vi "CheckForError.vi"(0 "Main Path":path) -> (1 "Array of Folders":path[](array[path]), 2 "PRAMMS VRN":refnum<visa-resource-name>, 3 "Array of Files":path[](array[path]), 4 "SkipInstr":bool, 6 "Bundle-Meteo":T1={"cRIO address"="0.0.0.0", "Port Number"=0, "cRIO_commID"=refnum, "Cx"=FALSE}, 8 "This VI's Path":path, 10 "term":string, 11 "Go on ?":bool, 12 "Array of Baud Rates":u32[](array[numeric]), 13 "TCS-CommVRN":refnum<visa-resource-name>, 14 "Array of VISA refnum":refnum<visa-resource-name>[](array[refnum]), 15 "Serial":bool[](array[boolean]))   [LabVIEW 2019]
uses:
  Globals.vi
  <vilib>/Utility/config.llb/Read Key (U32).vi
  <vilib>/Utility/config.llb/Read Key (String).vi
  <vilib>/Instr/_visa.llb/VISA Configure Serial Port (Instr).vi
  Comm/SerialCommError.vi
  <vilib>/Utility/config.llb/Read Key (Path).vi
  <vilib>/Utility/config.llb/NI_LVConfig.lvlib
panel:
  in  "SkipInstr":bool
  out "Hexapode":bool
  out "Hexapod VRN":refnum<visa-resource-name>
  out "PRAMMS":bool
  out "ActiveDummy":bool
  out "TCS":bool
  out "TCP Error":errorcluster
  out "standard output":string
  out "standard error":string
  out "concatenated string":string
  out "Nettoyage":bool
  in  "restart":bool
  out "error out":errorcluster
  in  "cancel":bool
  in  "ignore":bool
  out "Master Dir":path
  out "IDL":bool
  out "wget":bool
  out "Ports Series":bool
  out "SubVIs":bool
  out "config error out":errorcluster
  out "Camera":bool
  out "Starry Night":bool
  out "Configuration":bool
  out "Arborescence":bool
  # "Version sans GUI de ErrorCheck.vi  Vérifie :\n    - Existence des chemins/fichiers nécessaire\n    - Communication avec les différents périphériques\n    - Lien ActiveX avec Starry Night\n    - Vérifie la communication avec la station météo\n    - Vérifie l'état de la face avant des VIs utilisés\n    - Compatibilité des versions installées\n    - Vérifie la disponibilité des applications (wget, IDL)"
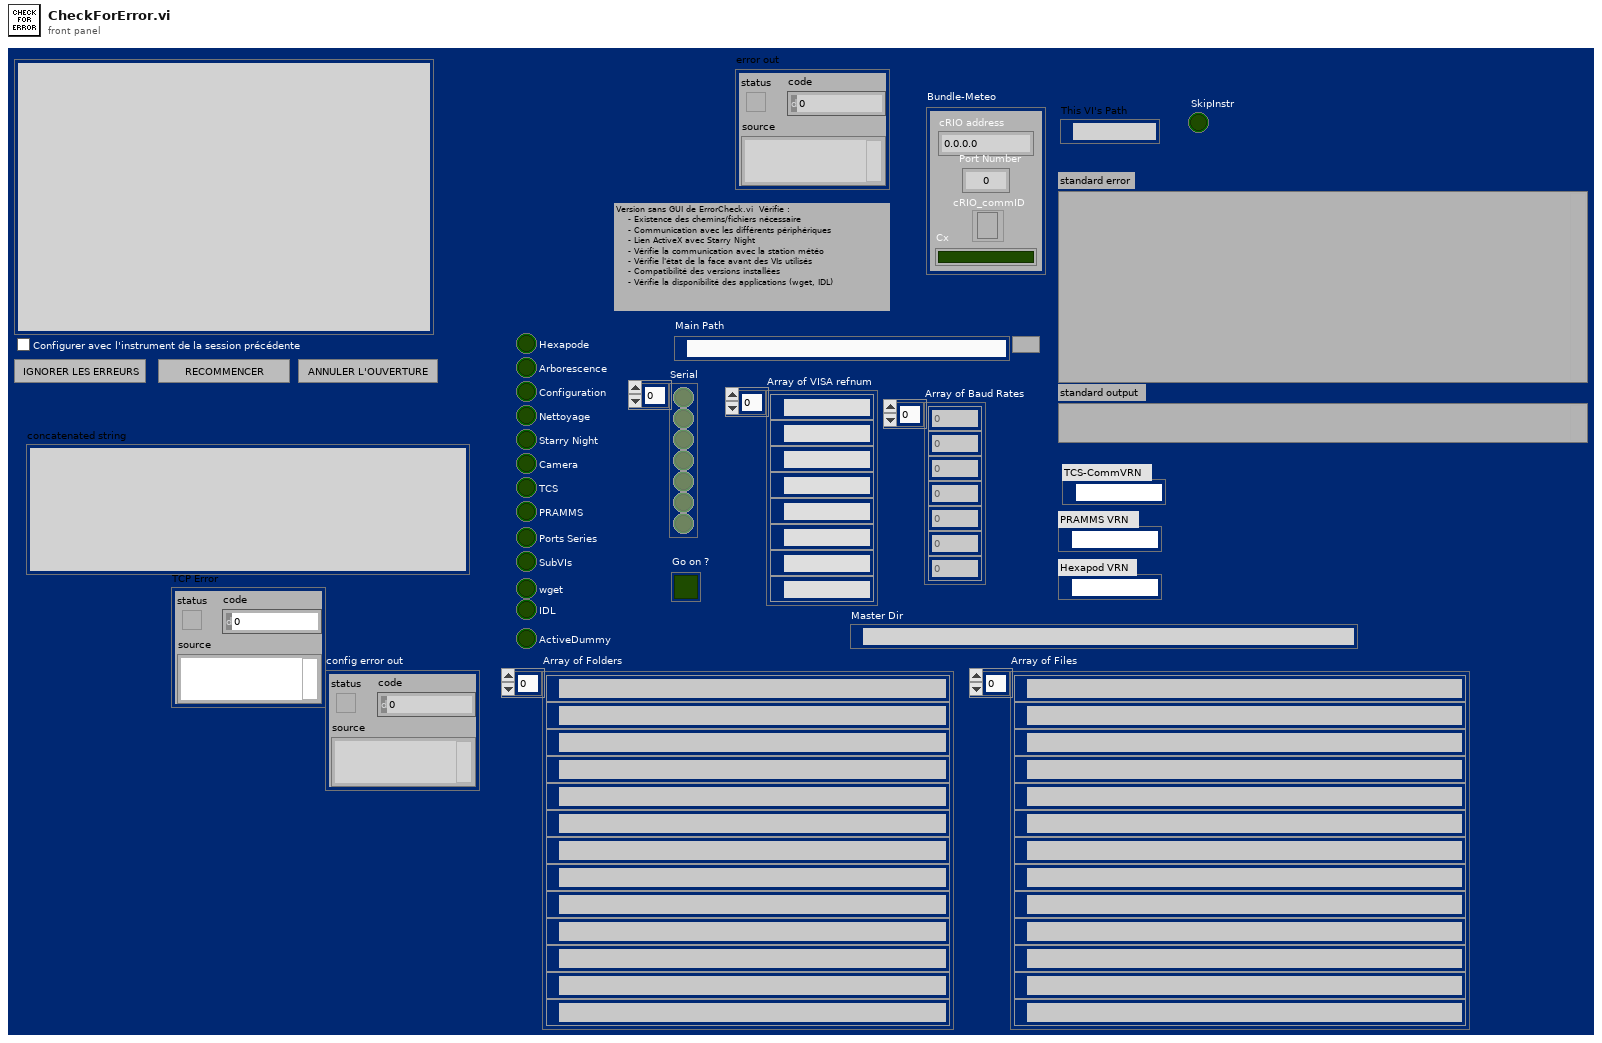
[diagram p1: front panel]
types:
  T1 = cluster{"cRIO address":string, "Port Number":u16, "cRIO_commID":refnum<k5>, "Cx":bool}
  T2 = enum8{"Enabled", "Disabled", "Disabled and Grayed Out"}
  T3 = typedef "NI_LVConfig.lvlib/Config Data RefNum.ctl" = refnum<k1>
  T4 = cluster{"value":string, u16, "connection ID":refnum<k5>, bool}
  T5 = enum16{"Left Button", "Center Button", "Right Button", "Window Close"}
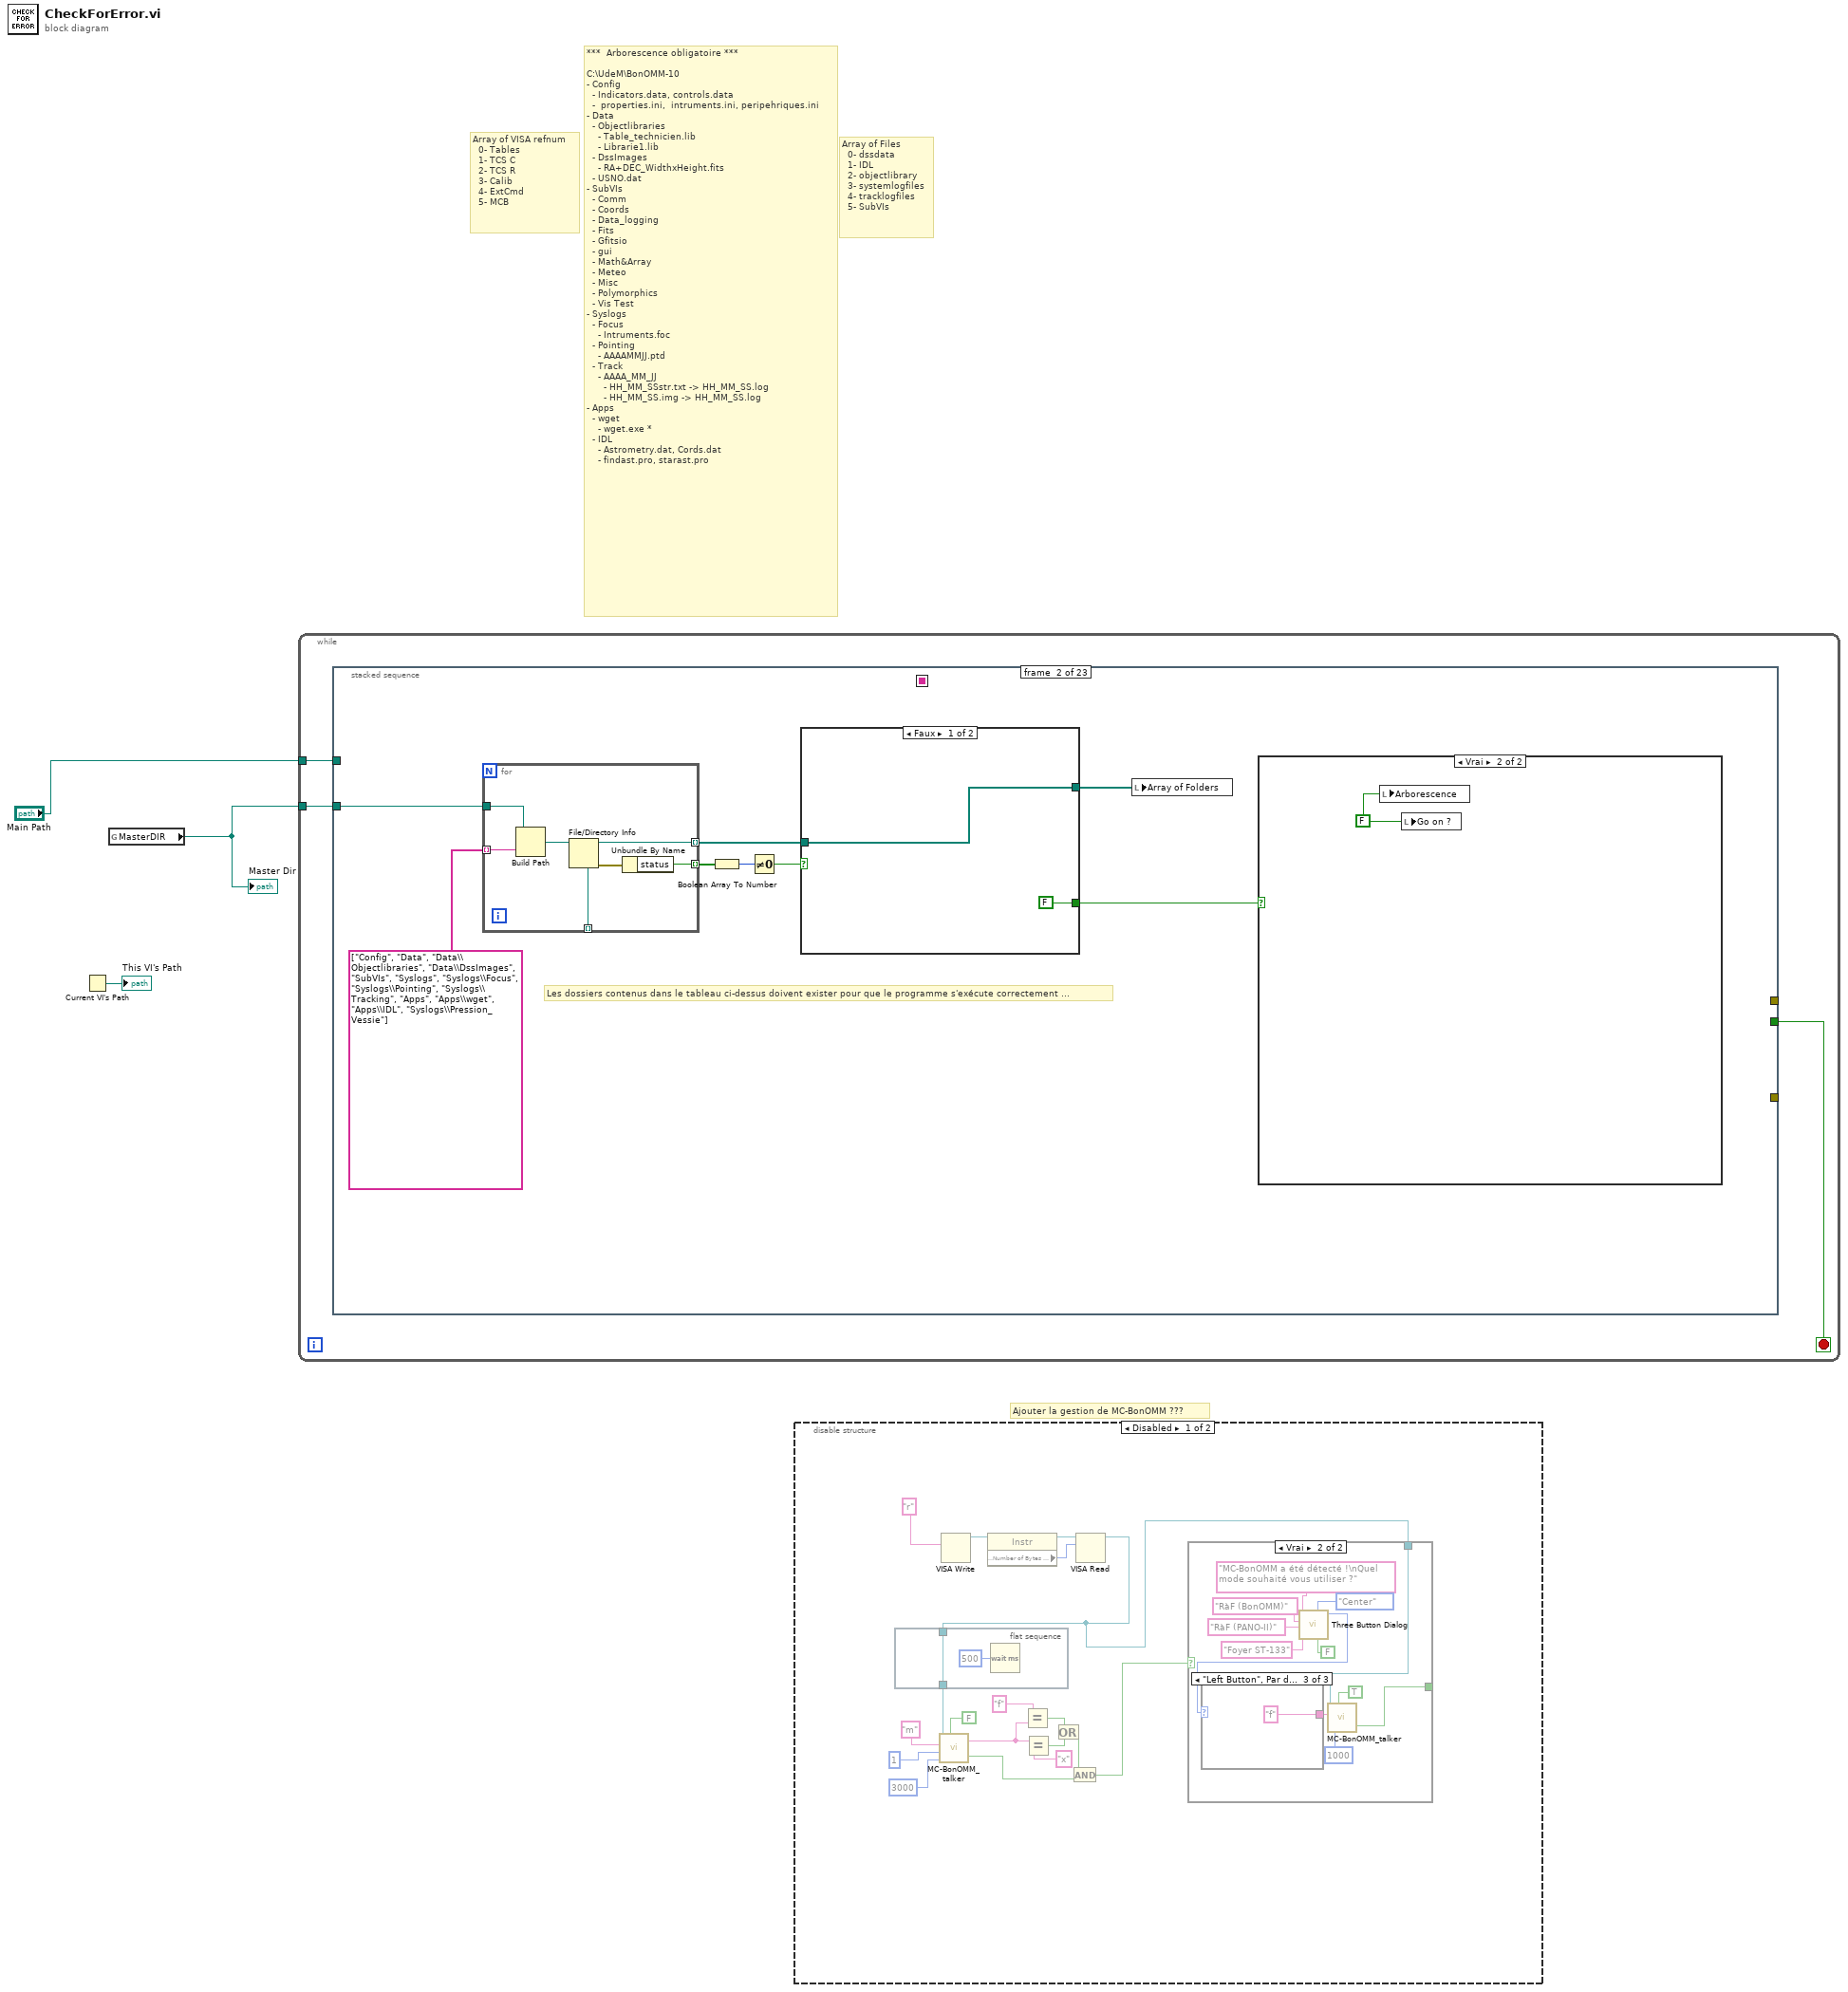
[diagram p0: block diagram]
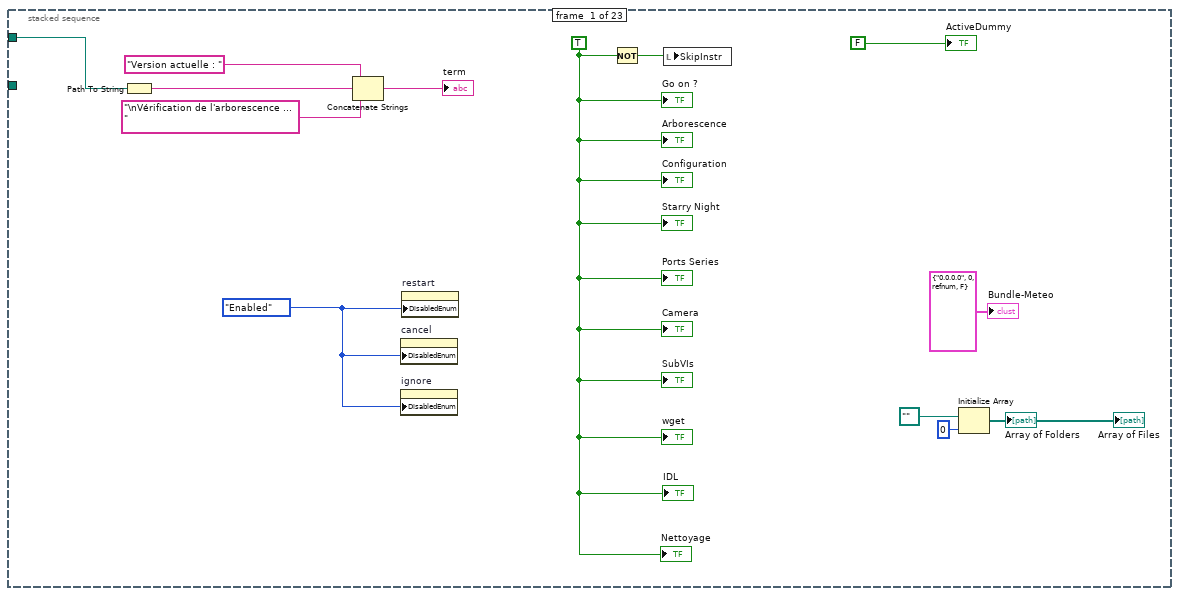
[diagram p2: hidden frame]
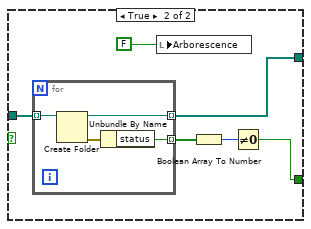
[diagram p4: hidden frame]
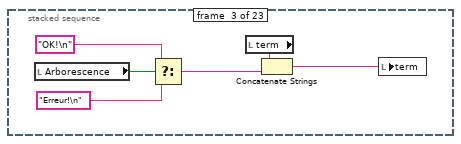
[diagram p5: hidden frame]
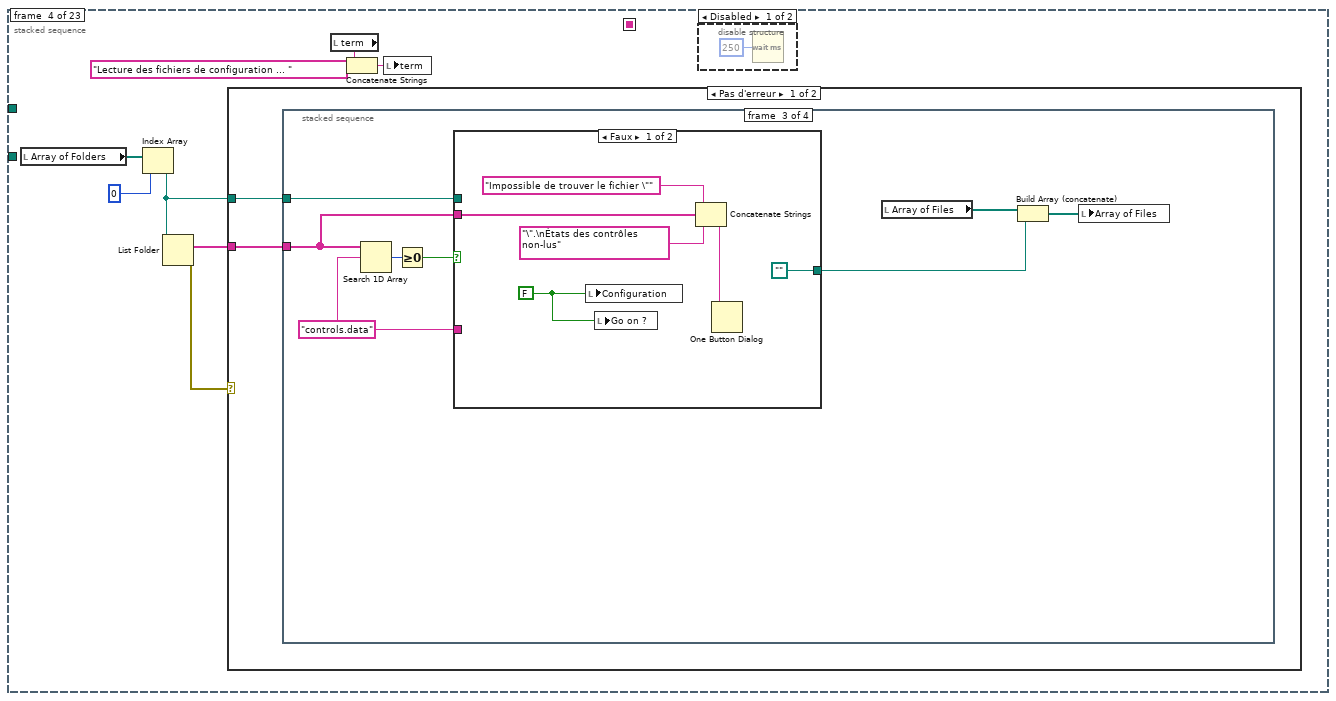
[diagram p6: hidden frame]
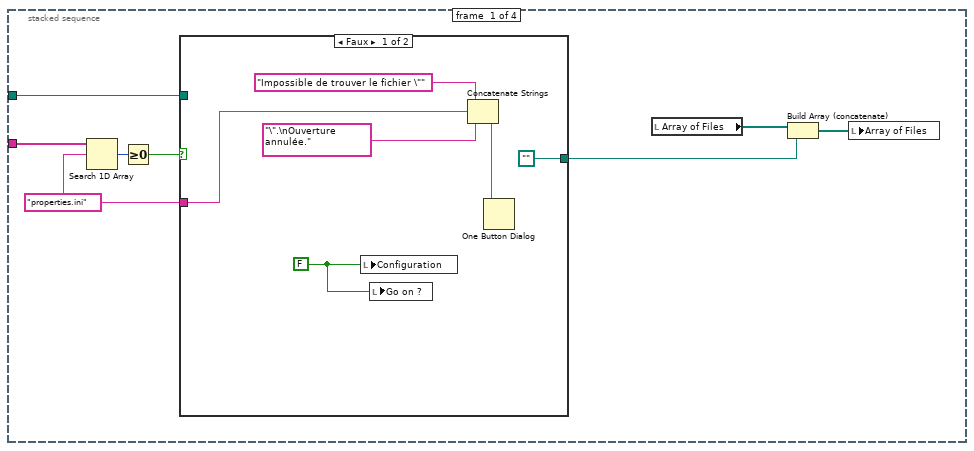
[diagram p8: hidden frame]
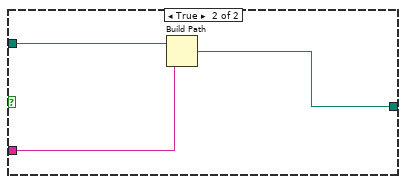
[diagram p9: hidden frame]
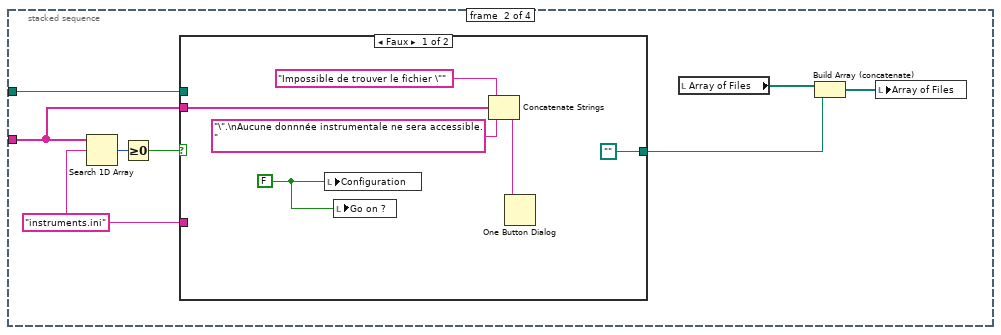
[diagram p10: hidden frame]
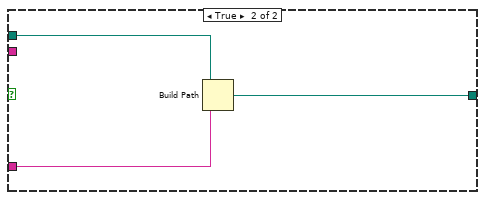
[diagram p11: hidden frame]
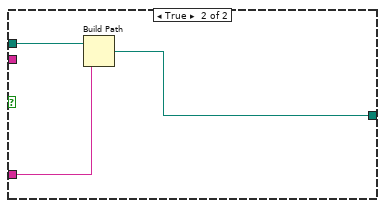
[diagram p12: hidden frame]
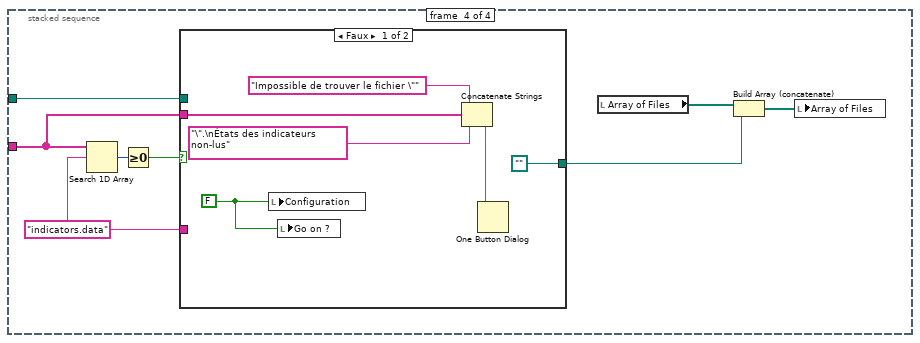
[diagram p13: hidden frame]
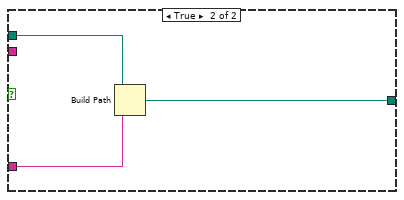
[diagram p14: hidden frame]
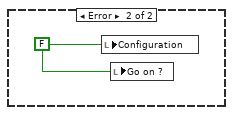
[diagram p15: hidden frame]
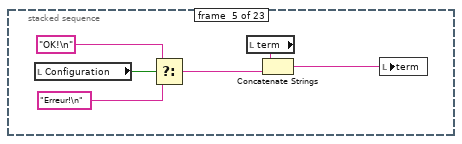
[diagram p16: hidden frame]
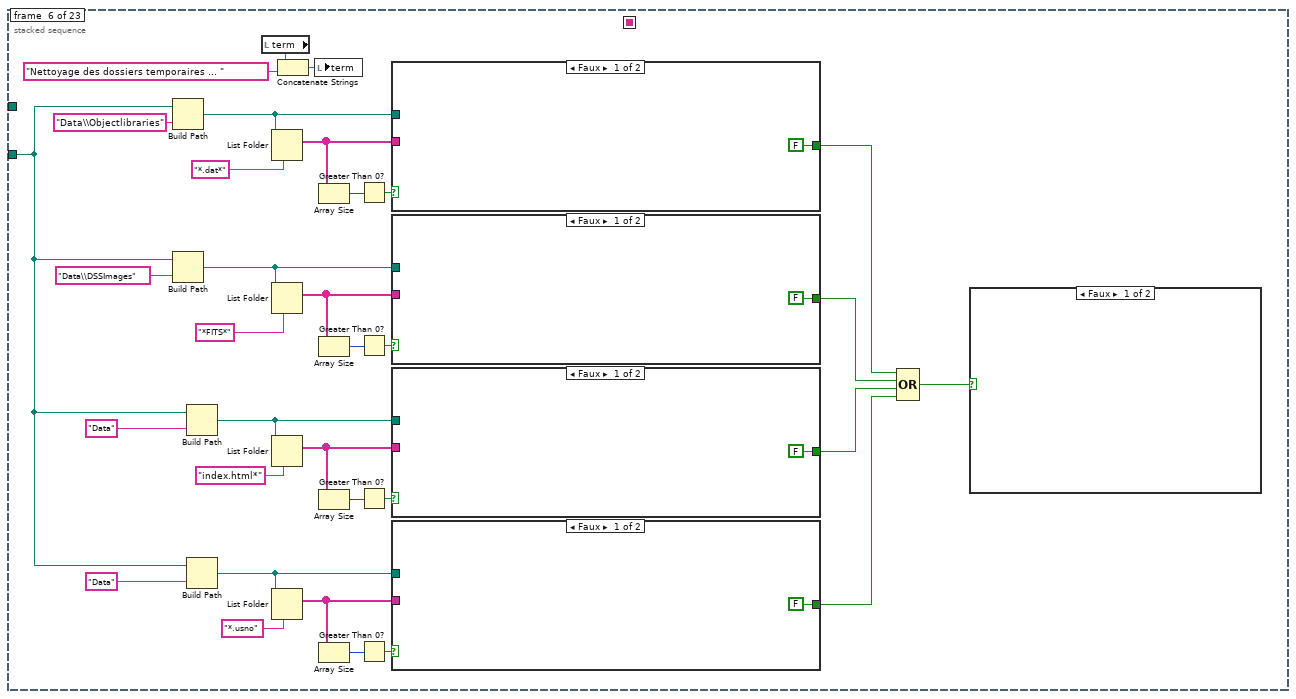
[diagram p17: hidden frame]
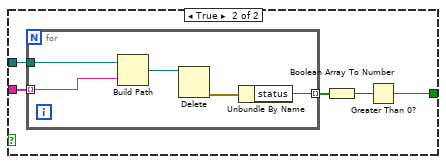
[diagram p18: hidden frame]
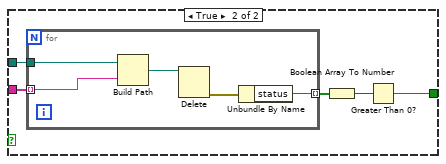
[diagram p19: hidden frame]
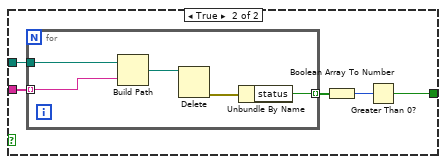
[diagram p20: hidden frame]
diagram:
  # "Array of Files\n  0- dssdata\n  1- IDL\n  2- objectlibrary\n  3- systemlogfiles\n  4- tracklogfiles\n  5- SubVIs"
  # "***  Arborescence obligatoire ***\n\nC:\\UdeM\\BonOMM-10\n-\tConfig\n  -\tIndicators.data, controls.data\n  -\t properties.ini,  intruments.ini, peripehriques.ini\n-\tData\n  -\tObjectlibraries\n    -\tTable_technicien.lib\n    -\tLibrarie1.lib\n  -\tDssImages\n    -\tRA+DEC_WidthxHeight.fits\n  -\tUSNO.dat\n-\tSubVIs\n  -\tComm\n  -\tCoords\n  -\tData_logging\n  -\tFits\n  -\tGfitsio\n  -\tgui\n  -\tMath&Array\n  -\tMeteo\n  -\tMisc\n  -\tPolymorphics\n  -\tVis Test\n-\tSyslogs\n  -\tFocus\n    -\tIntruments.foc\n  -\tPointing\n    -\tAAAAMMJJ.ptd\n  -\tTrack\n    -\tAAAA_MM_JJ\n      -\tHH_MM_SSstr.txt -> HH_MM_SS.log\n      -\tHH_MM_SS.img -> HH_MM_SS.log\n-\tApps\n  -\twget\n    -\twget.exe *\n  -\tIDL\n    -\tAstrometry.dat, Cords.dat\n    -\tfindast.pro, starast.pro"
  # "Array of VISA refnum\n  0- Tables\n  1- TCS C\n  2- TCS R\n  3- Calib\n  4- ExtCmd\n  5- MCB"
  # "Ajouter la gestion de MC-BonOMM ???"
  n1 = Current VI's Path() -> (path=→"This VI's Path":path)
  n2 = global read "Globals.vi" "MasterDIR"() -> (w1:path)
  "Master Dir" <- w1
  n3 = while {
    tunnel: w1 -> [w6]
    tunnel: "Main Path" -> [w5]
    stop <- w4 stop-if-true
    n4 = stacked-sequence {
      seq-local: [_ _ _ _ _ _ _ _ _ _ _ _ _ _ _ _ _ _ _ _ _ w680 _] -> [_ _ _ _ _ _ _ _ _ _ _ _ _ _ _ _ _ _ _ _ _ _ w718]
      tunnel: w6 -> [_ w26 _ _ _ w140 _ _ _ _ _ _ _ _ _ _ _ _ _ _ _ _ _]
      tunnel: w5 -> [w15 _ _ _ _ _ _ _ _ _ _ _ _ _ _ _ _ _ _ _ _ _ _]
      tunnel: [_ _ _ _ _ _ _ _ _ _ _ _ _ _ _ _ _ _ _ _ _ w681 _] -> w4
      tunnel: [_ _ _ _ _ _ _ _ _ _ _ _ _ _ w510 _ _ _ _ _ _ _ _] -> _
      tunnel: [_ _ _ _ _ _ _ _ _ _ _ _ w436 _ _ _ _ _ _ _ _ _ _] -> _
      frame #0 {
        w10 = T2."Enabled" ("Disabled")
        w7 = TRUE ("Arborescence")
        n5 = Path To String(path=w15) -> (string=w19:string)
        n6 = Concatenate Strings("Version actuelle : ", w19, "\nVérification de l'arborescence ... ") -> (→"term":string)
        n7 = property on="cancel" class="Bool"("DisabledEnum"=w10) -> ()  [unwired: 2 in, 2 out]
        n8 = property on="ignore" class="Bool"("DisabledEnum"=w10) -> ()  [unwired: 2 in, 2 out]
        n9 = property on="restart" class="Bool"("DisabledEnum"=w10) -> ()  [unwired: 2 in, 2 out]
        n10 = Not(x=w7) -> (.not. x?=w8:bool)
        n11 = local write "SkipInstr"(w8) -> ()
        n12 = Initialize Array(path "" ("path dup"), 0 ("dimension size")) -> (→"Array of Folders" →"Array of Files":path[])
        "Arborescence" <- w7
        "Go on ?" <- w7
        "Configuration" <- w7
        "Starry Night" <- w7
        "Camera" <- w7
        "SubVIs" <- w7
        "Ports Series" <- w7
        "wget" <- w7
        "IDL" <- w7
        "Bundle-Meteo" <- T1 {"cRIO address"="0.0.0.0", "Port Number"=0, "cRIO_commID"=refnum, "Cx"=FALSE} ("Bundle-Meteo")
        "Nettoyage" <- w7
        "ActiveDummy" <- FALSE ("Arborescence")
      }
      frame #1 {
        # "Les dossiers contenus dans le tableau ci-dessus doivent exister pour que le programme s'exécute correctement ..."
        n13 = for {
          tunnel: string[] ["Config", "Data", "Data\\Objectlibraries", "Data\\DssImages", "SubVIs", "Syslogs", "Syslogs\\Focus", "Syslogs\\Pointing", "Syslogs\\Tracking", "Apps", "Apps\\wget", "Apps\\IDL", "Syslogs\\Pression_Vessie"] -> [w46] mode=indexing
          tunnel: w26 -> [w47]
          tunnel: [w44] -> w22 mode=indexing
          tunnel: [w43] -> _ mode=indexing
          tunnel: [w41] -> w25 mode=indexing
          n14 = Build Path(base path=w47, name or relative path=w46) -> (appended path=w45:path)
          n15 = File/Directory Info(path=w45) -> (path out=w44:path, error out=w42:errorcluster, resolved path=w43:path)  [unwired: 1 in, 4 out]
          n16 = Unbundle By Name(w42) -> ("status"=w41:bool)
        }
        n17 = Boolean Array To Number(Boolean array=w25) -> (number=w24:u32)
        n18 = Not Equal To 0?(x=w24) -> (x != 0?=w23:bool)
        n19 = case shown="Faux" w23 {
          tunnel: w22 -> [w29 w36]
          tunnel: [FALSE w33] -> w21
          tunnel: [w29 w32] -> w20
          frame False {
          }
          frame True {
            n20 = for {
              tunnel: w36 -> [w40] mode=indexing
              tunnel: [w38] -> w34 mode=indexing
              tunnel: [w37] -> w32 mode=indexing
              n21 = Create Folder(path (use dialog)=w40) -> (created path=w37:path, error out=w39:errorcluster)  [unwired: 2 in, 1 out]
              n22 = Unbundle By Name(w39) -> ("status"=w38:bool)
            }
            n23 = local write "Arborescence"(FALSE) -> ()
            n24 = Boolean Array To Number(Boolean array=w34) -> (number=w35:u32)
            n25 = Not Equal To 0?(x=w35) -> (x != 0?=w33:bool)
          }
        }
        n26 = local write "Array of Folders"(w20) -> ()
        n27 = case shown="Vrai" w21 {
          frame False {
          }
          frame True {
            w28 = FALSE
            n28 = local write "Arborescence"(w28) -> ()
            n29 = local write "Go on ?"(w28) -> ()
          }
        }
      }
      frame #2 {
        n30 = local read "Arborescence"() -> (w50:bool)
        n31 = Select(t="OK!\n" ("string"), s=w50, f="Erreur!\n" ("string")) -> (s? t:f=w51:string)
        n32 = local read "term"() -> (w52:string)
        n33 = Concatenate Strings(w52, w51) -> (w53:string)
        n34 = local write "term"(w53) -> ()
      }
      frame #3 {
        n35 = local read "Array of Folders"() -> (w56:path[])
        n36 = Index Array(array=w56, index=0) -> (element=w54:path)
        n37 = List Folder(path=w54) -> (filenames=w58:string[], error out=w57:errorcluster)  [unwired: 3 in, 2 out]
        n38 = case shown="Pas d'erreur" w57 {
          tunnel: w58 -> [w64 _]
          tunnel: w54 -> [w63 _]
          frame No Error {
            n39 = stacked-sequence {
              tunnel: w64 -> [w70 w87 w104 w121]
              tunnel: w63 -> [w67 w85 w103 w120]
              frame #0 {
                w66 = "properties.ini"
                n40 = Search 1D Array(1D array=w70, element=w66) -> (index of element=w72:i32)  [unwired: 1 in]
                n41 = Greater Or Equal To 0?(x=w72) -> (x >= 0?=w71:bool)
                n42 = case shown="Faux" w71 {
                  tunnel: w67 -> [_ w81]
                  tunnel: w66 -> [w74 w80]
                  tunnel: [path "" w79] -> w65
                  frame False {
                    w75 = FALSE ("Configuration")
                    n43 = local write "Configuration"(w75) -> ()
                    n44 = local write "Go on ?"(w75) -> ()
                    n45 = Concatenate Strings("Impossible de trouver le fichier \"", w74, "\".\nOuverture annulée.") -> (w76:string)
                    n46 = One Button Dialog(message=w76) -> ()  [unwired: 1 in, 1 out]
                  }
                  frame True {
                    n47 = Build Path(base path=w81, name or relative path=w80) -> (appended path=w79:path)
                  }
                }
                n48 = local read "Array of Files"() -> (w69:path[])
                n49 = Build Array (concatenate)(w69, w65) -> (w68:path[])
                n50 = local write "Array of Files"(w68) -> ()
              }
              frame #1 {
                w86 = "instruments.ini"
                n51 = Search 1D Array(1D array=w87, element=w86) -> (index of element=w89:i32)  [unwired: 1 in]
                n52 = Greater Or Equal To 0?(x=w89) -> (x >= 0?=w88:bool)
                n53 = case shown="Faux" w88 {
                  tunnel: w87 -> [w93 _]
                  tunnel: w86 -> [_ w98]
                  tunnel: w85 -> [_ w97]
                  tunnel: [path "" w96] -> w82
                  frame False {
                    w91 = FALSE ("Configuration")
                    n54 = local write "Configuration"(w91) -> ()
                    n55 = local write "Go on ?"(w91) -> ()
                    n56 = Concatenate Strings("Impossible de trouver le fichier \"", w93, "\".\nAucune donnnée instrumentale ne sera accessible.") -> (w92:string)
                    n57 = One Button Dialog(message=w92) -> ()  [unwired: 1 in, 1 out]
                  }
                  frame True {
                    n58 = Build Path(base path=w97, name or relative path=w98) -> (appended path=w96:path)
                  }
                }
                n59 = local read "Array of Files"() -> (w84:path[])
                n60 = Build Array (concatenate)(w84, w82) -> (w83:path[])
                n61 = local write "Array of Files"(w83) -> ()
              }
              frame #2 {
                w102 = "controls.data"
                n62 = Search 1D Array(1D array=w104, element=w102) -> (index of element=w106:i32)  [unwired: 1 in]
                n63 = Greater Or Equal To 0?(x=w106) -> (x >= 0?=w105:bool)
                n64 = case shown="Faux" w105 {
                  tunnel: w104 -> [w110 _]
                  tunnel: w103 -> [_ w115]
                  tunnel: w102 -> [_ w114]
                  tunnel: [path "" w113] -> w99
                  frame False {
                    w108 = FALSE ("Configuration")
                    n65 = local write "Configuration"(w108) -> ()
                    n66 = local write "Go on ?"(w108) -> ()
                    n67 = Concatenate Strings("Impossible de trouver le fichier \"", w110, "\".\nÉtats des contrôles non-lus") -> (w109:string)
                    n68 = One Button Dialog(message=w109) -> ()  [unwired: 1 in, 1 out]
                  }
                  frame True {
                    n69 = Build Path(base path=w115, name or relative path=w114) -> (appended path=w113:path)
                  }
                }
                n70 = local read "Array of Files"() -> (w101:path[])
                n71 = Build Array (concatenate)(w101, w99) -> (w100:path[])
                n72 = local write "Array of Files"(w100) -> ()
              }
              frame #3 {
                w119 = "indicators.data"
                n73 = Search 1D Array(1D array=w121, element=w119) -> (index of element=w123:i32)  [unwired: 1 in]
                n74 = Greater Or Equal To 0?(x=w123) -> (x >= 0?=w122:bool)
                n75 = case shown="Faux" w122 {
                  tunnel: w121 -> [w127 _]
                  tunnel: w120 -> [_ w132]
                  tunnel: w119 -> [_ w131]
                  tunnel: [path "" w130] -> w116
                  frame False {
                    w125 = FALSE ("Configuration")
                    n76 = local write "Configuration"(w125) -> ()
                    n77 = local write "Go on ?"(w125) -> ()
                    n78 = Concatenate Strings("Impossible de trouver le fichier \"", w127, "\".\nÉtats des indicateurs non-lus") -> (w126:string)
                    n79 = One Button Dialog(message=w126) -> ()  [unwired: 1 in, 1 out]
                  }
                  frame True {
                    n80 = Build Path(base path=w132, name or relative path=w131) -> (appended path=w130:path)
                  }
                }
                n81 = local read "Array of Files"() -> (w118:path[])
                n82 = Build Array (concatenate)(w118, w116) -> (w117:path[])
                n83 = local write "Array of Files"(w117) -> ()
              }
            }
          }
          frame Error {
            w133 = FALSE ("Configuration")
            n84 = local write "Configuration"(w133) -> ()
            n85 = local write "Go on ?"(w133) -> ()
          }
        }
        n86 = local read "term"() -> (w60:string)
        n87 = Concatenate Strings(w60, "Lecture des fichiers de configuration ... " ("string")) -> (w61:string)
        n88 = local write "term"(w61) -> ()
        n89 = disable-structure shown="Disabled" {
          frame Disabled {
            n90 = Wait (ms)(milliseconds to wait=u32 250) -> ()  [unwired: 1 out]
          }
          frame Enabled {
          }
        }
      }
      frame #4 {
        n91 = local read "Configuration"() -> (w136:bool)
        n92 = Select(t="OK!\n" ("string"), s=w136, f="Erreur!\n" ("string")) -> (s? t:f=w137:string)
        n93 = local read "term"() -> (w138:string)
        n94 = Concatenate Strings(w138, w137) -> (w139:string)
        n95 = local write "term"(w139) -> ()
      }
      frame #5 {
        n96 = Build Path(base path=w140, name or relative path="Data\\Objectlibraries") -> (appended path=w165:path)
        n97 = Build Path(base path=w140, name or relative path="Data\\DSSImages") -> (appended path=w163:path)
        n98 = Build Path(base path=w140, name or relative path="Data") -> (appended path=w149:path)
        n99 = Build Path(base path=w140, name or relative path="Data") -> (appended path=w146:path)
        n100 = local read "term"() -> (w171:string)
        n101 = List Folder(path=w165, pattern="*.dat*") -> (filenames=w167:string[])  [unwired: 2 in, 3 out]
        n102 = List Folder(path=w163, pattern="*FITS*") -> (filenames=w161:string[])  [unwired: 2 in, 3 out]
        n103 = List Folder(path=w149, pattern="index.html*") -> (filenames=w151:string[])  [unwired: 2 in, 3 out]
        n104 = List Folder(path=w146, pattern="*.usno") -> (filenames=w145:string[])  [unwired: 2 in, 3 out]
        n105 = Concatenate Strings(w171, "Nettoyage des dossiers temporaires ... " ("string")) -> (w172:string)
        n106 = local write "term"(w172) -> ()
        n107 = Array Size(array=w167) -> (size(s)=w168:i32)
        n108 = Array Size(array=w161) -> (size(s)=w160:i32)
        n109 = Array Size(array=w151) -> (size(s)=w152:i32)
        n110 = Array Size(array=w145) -> (size(s)=w144:i32)
        n111 = Greater Than 0?(x=w168) -> (x > 0?=w169:bool)
        n112 = Greater Than 0?(x=w160) -> (x > 0?=w159:bool)
        n113 = Greater Than 0?(x=w152) -> (x > 0?=w153:bool)
        n114 = Greater Than 0?(x=w144) -> (x > 0?=w143:bool)
        n115 = case shown="Faux" w169 {
          tunnel: w167 -> [_ w211]
          tunnel: w165 -> [_ w210]
          tunnel: [FALSE w207] -> w157
          frame False {
          }
          frame True {
            n116 = for {
              tunnel: w211 -> [w215] mode=indexing
              tunnel: w210 -> [w216]
              tunnel: [w212] -> w209 mode=indexing
              n117 = Build Path(base path=w216, name or relative path=w215) -> (appended path=w214:path)
              n118 = Delete(path (use dialog)=w214) -> (error out=w213:errorcluster)  [unwired: 4 in, 2 out]
              n119 = Unbundle By Name(w213) -> ("status"=w212:bool)
            }
            n120 = Boolean Array To Number(Boolean array=w209) -> (number=w208:u32)
            n121 = Greater Than 0?(x=w208) -> (x > 0?=w207:bool)
          }
        }
        n122 = case shown="Faux" w159 {
          tunnel: w161 -> [_ w200]
          tunnel: w163 -> [_ w199]
          tunnel: [FALSE w196] -> w156
          frame False {
          }
          frame True {
            n123 = for {
              tunnel: w200 -> [w204] mode=indexing
              tunnel: w199 -> [w205]
              tunnel: [w201] -> w198 mode=indexing
              n124 = Build Path(base path=w205, name or relative path=w204) -> (appended path=w203:path)
              n125 = Delete(path (use dialog)=w203) -> (error out=w202:errorcluster)  [unwired: 4 in, 2 out]
              n126 = Unbundle By Name(w202) -> ("status"=w201:bool)
            }
            n127 = Boolean Array To Number(Boolean array=w198) -> (number=w197:u32)
            n128 = Greater Than 0?(x=w197) -> (x > 0?=w196:bool)
          }
        }
        n129 = case shown="Faux" w153 {
          tunnel: w151 -> [_ w189]
          tunnel: w149 -> [_ w188]
          tunnel: [FALSE w185] -> w150
          frame False {
          }
          frame True {
            n130 = for {
              tunnel: w189 -> [w193] mode=indexing
              tunnel: w188 -> [w194]
              tunnel: [w190] -> w187 mode=indexing
              n131 = Build Path(base path=w194, name or relative path=w193) -> (appended path=w192:path)
              n132 = Delete(path (use dialog)=w192) -> (error out=w191:errorcluster)  [unwired: 4 in, 2 out]
              n133 = Unbundle By Name(w191) -> ("status"=w190:bool)
            }
            n134 = Boolean Array To Number(Boolean array=w187) -> (number=w186:u32)
            n135 = Greater Than 0?(x=w186) -> (x > 0?=w185:bool)
          }
        }
        n136 = case shown="Faux" w143 {
          tunnel: w145 -> [_ w178]
          tunnel: w146 -> [_ w177]
          tunnel: [FALSE w174] -> w141
          frame False {
          }
          frame True {
            n137 = for {
              tunnel: w178 -> [w182] mode=indexing
              tunnel: w177 -> [w183]
              tunnel: [w179] -> w176 mode=indexing
              n138 = Build Path(base path=w183, name or relative path=w182) -> (appended path=w181:path)
              n139 = Delete(path (use dialog)=w181) -> (error out=w180:errorcluster)  [unwired: 4 in, 2 out]
              n140 = Unbundle By Name(w180) -> ("status"=w179:bool)
            }
            n141 = Boolean Array To Number(Boolean array=w176) -> (number=w175:u32)
            n142 = Greater Than 0?(x=w175) -> (x > 0?=w174:bool)
          }
        }
        n143 = Compound Arithmetic op=OR(w157, w156, w150, w141) -> (w158:bool)
        n144 = case shown="Faux" w158 {
          frame False {
          }
          frame True {
            w217 = FALSE
            n145 = local write "Nettoyage"(w217) -> ()
            n146 = local write "Go on ?"(w217) -> ()
          }
        }
      }
      frame #6 {
        n147 = local read "Nettoyage"() -> (w220:bool)
        n148 = Select(t="OK!\n" ("string"), s=w220, f="Erreur!\n" ("string")) -> (s? t:f=w221:string)
        n149 = local read "term"() -> (w222:string)
        n150 = Concatenate Strings(w222, w221) -> (w223:string)
        n151 = local write "term"(w223) -> ()
      }
      frame #7 {
        n152 = local read "term"() -> (w230:string)
        n153 = Concatenate Strings(w230, "Test du lien ActiveX avec Starry Night ... " ("string")) -> (w231:string)
        n154 = local write "term"(w231) -> ()
        n155 = Automation Open(Automation Refnum=refnum<k7> refnum ("ScopeSim._Telescope")) -> (Automation Refnum=w224:refnum<k7>, error out=w227:errorcluster)  [unwired: 3 in]
        n156 = Unbundle By Name(w227) -> ("status"=w226:bool)
        n157 = case shown="Vrai" w226 {
          tunnel: w224 -> [w234 _]
          tunnel: [w233 FALSE ("Connected")] -> w228
          frame False {
            n158 = property class="_Telescope"(reference=w234) -> (reference out=w232:refnum<k7>, "Connected"=w233:bool)  [unwired: 1 in, 1 out]
            n159 = Close Reference(reference=w232) -> ()  [unwired: 1 in, 1 out]
          }
          frame True {
          }
        }
        n160 = global write "Globals.vi" "ScopeSim._Telescope"(w224) -> ()
        n161 = case shown="Vrai" w228 {
          frame False {
            w236 = FALSE
            n162 = local write "Starry Night"(w236) -> ()
            n163 = local write "Go on ?"(w236) -> ()
          }
          frame True {
          }
        }
      }
      frame #8 {
        n164 = local read "Starry Night"() -> (w237:bool)
        n165 = Select(t="OK!\n" ("string"), s=w237, f="Erreur!\n" ("string")) -> (s? t:f=w240:string)
        n166 = local read "term"() -> (w241:string)
        n167 = Concatenate Strings(w241, w240) -> (w242:string)
        n168 = local write "term"(w242) -> ()
      }
      frame #9 {
        n169 = local read "Array of Files"() -> (w245:path[])
        n170 = Index Array(array=w245, index=0) -> (element=w244:path)
        n171 = call <vilib>:"Open Config Data.vi"("configuration file path"=w244) -> ("error out"=w253:errorcluster, "refnum"=w255:T3)  [unwired: 8 in, 1 out]
        n172 = for {
          tunnel: string[] ["tablespd", "calibspd", "excspd", "mcbspd", "splspd"] -> [w276] mode=indexing
          tunnel: string[] ["tablevrn", "calibvrn", "excvrn", "mcbvrn", "splvrn"] -> [w275] mode=indexing
          tunnel: "communications" -> [w268]
          tunnel: w255 -> [w278]
          tunnel: [w277] -> w254
          shift-right: [w273] -> w252
          shift-left: w253 -> [w274]
          tunnel: [w265] -> w248 mode=indexing
          tunnel: [w267] -> w247 mode=indexing
          tunnel: [w261] -> w246 mode=indexing
          tunnel: [w263] -> _ mode=indexing
          i -> [w269]
          n173 = call-poly <vilib>:"Read Key.vi"("section"=w268, "error in (no error)"=w274, "default value"=u32 9600, "key"=w276, "refnum"=w278) -> ("error out"=w279:errorcluster, "value"=w261:u32, "refnum out"=w280:T3)  [unwired: 3 in, 1 out]
          n174 = call-poly <vilib>:"Read Key.vi"("section"=w268, "error in (no error)"=w279, "default value"="-1", "key"=w275, "refnum"=w280) -> ("error out"=w273:errorcluster, "value"=w264:string, "refnum out"=w277:T3)  [unwired: 3 in, 1 out]
          n175 = Type Cast(type=refnum<visa-resource-name> "-1" ("Table VRN"), x=w264) -> (*(type *) &x=w262:refnum<visa-resource-name>)
          n176 = case shown="0" w269 {
            tunnel: w262 -> [_ w309 w318 w339 w355 w376]
            tunnel: [refnum<visa-resource-name> "-1" ("Table VRN") w301 w330 w337 w353 w373] -> w266
            tunnel: [FALSE ("ok ?") w305 w331 w349 w360 w375] -> w267
            tunnel: w264 -> [_ w313 w325 w344 w361 w372]
            tunnel: w261 -> [_ w303 w320 w338 w354 w367]
            tunnel: [errorcluster {"status"=FALSE, "code"=0, "source"=""} ("error out") w298 w317 w336 w352 w374] -> w260
            frame -1, Default {
              (unwired) "Bizzarerie ... " ("string")
            }
            frame 0 {
              n177 = control-ref of="ActiveDummy"() -> (w297:refnum<vi>)
              n178 = Equal?(x=refnum<visa-resource-name> "N/A" ("Table VRN"), y=w309) -> (x = y?=w307:bool)
              n179 = Select(t=refnum<visa-resource-name> "-1", s=w307, f=w309) -> (s? t:f=w304:refnum<visa-resource-name>)
              n180 = call "Newmark-Initialize.vi"("VISA resource name"=w304, "ActiveStages"=string[] ["AX", "AY", "AZ"], "baud rate"=w303, "Timeout"=u32 1000, "Bool Refnum"=w297) -> ("VISA resource name out"=w301:refnum<visa-resource-name>, "Error?"=w300:bool, "Error OUT"=w298:errorcluster)  [unwired: 8 in]
              n181 = Not(x=w307) -> (.not. x?=w308:bool)
              n182 = local read "term"() -> (w316:string)
              n183 = Concatenate Strings(w316, "   Table de guidage (" ("string"), w313, ") ... " ("string")) -> (w315:string)
              n184 = And(x=w300, y=w308) -> (x .and. y?=w306:bool)
              n185 = Not(x=w306) -> (.not. x?=w305:bool)
              n186 = local write "term"(w315) -> ()
            }
            frame 1 {
              w324 = u16 0 items=["None", "XON/XOFF", "RTS/CTS", "XON/XOFF & RTS/CTS", "DTR/DSR", "XON/XOFF & DTR/DSR"] ("flow control (0:none)")
              w323 = u16 10 items=["1.0"=10, "1.5"=15, "2.0"=20] ("stop bits (10: 1 bit)")
              n187 = call-poly "VISA Configure Serial Port"("VISA resource name"=w318, "baud rate (9600)"=w320, "data bits (8)"=u16 8, "parity (0:none)"=enum16{"None", "Odd", "Even", "Mark", "Space"}."None", "stop bits (10: 1 bit)"=w323, "flow control (0:none)"=w324) -> ("VISA resource name out"=w319:refnum<visa-resource-name>, "error out"=w317:errorcluster)  [unwired: 8 in]
              n188 = call "Controle_des_lampe.vi"("VISA resource name"=w319, "Status In"=bool[] [FALSE, FALSE, FALSE]) -> ("VISA resource name dup"=w330:refnum<visa-resource-name>, "Status Out"=w334:bool[])  [unwired: 1 out]
              n189 = local read "term"() -> (w329:string)
              n190 = Concatenate Strings(w329, "   Module de caibration (" ("string"), w325, ") ... " ("string")) -> (w328:string)
              n191 = Boolean Array To Number(Boolean array=w334) -> (number=w332:u32)
              n192 = Equal To 0?(x=w332) -> (x = 0?=w331:bool)
              n193 = local write "term"(w328) -> ()
            }
            frame 2 {
              w343 = u16 0 items=["None", "XON/XOFF", "RTS/CTS", "XON/XOFF & RTS/CTS", "DTR/DSR", "XON/XOFF & DTR/DSR"] ("flow control (0:none)")
              w342 = u16 10 items=["1.0"=10, "1.5"=15, "2.0"=20] ("stop bits (10: 1 bit)")
              n194 = call-poly "VISA Configure Serial Port"("VISA resource name"=w339, "Enable Termination\nChar (T)"=FALSE ("Enable Termination\nChar (T)"), "baud rate (9600)"=w338, "data bits (8)"=u16 8, "parity (0:none)"=enum16{"None", "Odd", "Even", "Mark", "Space"}."None", "stop bits (10: 1 bit)"=w342, "flow control (0:none)"=w343) -> ("VISA resource name out"=w337:refnum<visa-resource-name>, "error out"=w336:errorcluster)  [unwired: 7 in]
              n195 = local read "term"() -> (w348:string)
              n196 = Concatenate Strings(w348, "   Commandes Externes (" ("string"), w344, ") ... " ("string")) -> (w347:string)
              n197 = Unbundle By Name(w336) -> ("status"=w350:bool)
              n198 = local write "term"(w347) -> ()
              n199 = Not(x=w350) -> (.not. x?=w349:bool)
            }
            frame 3 {
              w359 = u16 0 items=["None", "XON/XOFF", "RTS/CTS", "XON/XOFF & RTS/CTS", "DTR/DSR", "XON/XOFF & DTR/DSR"] ("flow control (0:none)")
              w358 = u16 10 items=["1.0"=10, "1.5"=15, "2.0"=20] ("stop bits (10: 1 bit)")
              n200 = call-poly "VISA Configure Serial Port"("VISA resource name"=w355, "Enable Termination\nChar (T)"=FALSE ("Enable Termination\nChar (T)"), "baud rate (9600)"=w354, "data bits (8)"=u16 8, "parity (0:none)"=enum16{"None", "Odd", "Even", "Mark", "Space"}."None", "stop bits (10: 1 bit)"=w358, "flow control (0:none)"=w359) -> ("VISA resource name out"=w353:refnum<visa-resource-name>, "error out"=w352:errorcluster)  [unwired: 7 in]
              n201 = local read "term"() -> (w365:string)
              n202 = Concatenate Strings(w365, "   MC-BonOMM (" ("string"), w361, ") ... " ("string")) -> (w364:string)
              n203 = Unbundle By Name(w352) -> ("status"=w366:bool)
              n204 = local write "term"(w364) -> ()
              n205 = Not(x=w366) -> (.not. x?=w360:bool)
            }
            frame 4 {
              n206 = disable-structure shown="Enabled" {
                disable-tunnel: w376 -> [w381 w385]
                disable-tunnel: [w380 w389] -> w375
                disable-tunnel: [w379 w384] -> w374
                disable-tunnel: [w378 w386] -> w373
                disable-tunnel: w367 -> [_ w383]
                frame Disabled {
                  n207 = call "MicroSlide-Initialize.vi"("VISA resource name"=w381) -> ("VRN OUT"=w378:refnum<visa-resource-name>, "Error OUT"=w379:errorcluster)  [unwired: 13 in]
                  n208 = Unbundle By Name(w379) -> ("status"=w377:bool)
                  n209 = Not(x=w377) -> (.not. x?=w380:bool)
                }
                frame Enabled {
                  n210 = call-poly "VISA Configure Serial Port"("VISA resource name"=w385, "timeout (10sec)"=u32 1000, "Enable Termination\nChar (T)"=FALSE ("Enable Termination\nChar (T)"), "baud rate (9600)"=w383) -> ("VISA resource name out"=w386:refnum<visa-resource-name>, "error out"=w384:errorcluster)  [unwired: 10 in]
                  n211 = Unbundle By Name(w384) -> ("status"=w388:bool)
                  n212 = Not(x=w388) -> (.not. x?=w389:bool)
                }
              }
              n213 = local read "term"() -> (w371:string)
              n214 = Concatenate Strings(w371, "   Lame séparatrice (" ("string"), w372, ") ... " ("string")) -> (w370:string)
              n215 = local write "term"(w370) -> ()
            }
          }
          n216 = case shown="Vrai" w267 {
            tunnel: w266 -> [w284 w291]
            tunnel: [refnum<visa-resource-name> "-1" ("VISA resource name out") w291] -> w265
            tunnel: [w282 w289] -> w263
            tunnel: w260 -> [w281 w289]
            frame False {
              w283 = FALSE ("Ports Series")
              n217 = local read "term"() -> (w287:string)
              n218 = VISA Close(VISA resource name=w284, error in (no error)=w281) -> (error out=w282:errorcluster)
              n219 = local write "Ports Series"(w283) -> ()
              n220 = Concatenate Strings(w287, "Erreur!\n" ("string")) -> (w286:string)
              n221 = local write "Go on ?"(w283) -> ()
              n222 = local write "term"(w286) -> ()
            }
            frame True {
              n223 = local read "term"() -> (w293:string)
              n224 = Concatenate Strings(w293, "OK!\n" ("string")) -> (w292:string)
              n225 = local write "term"(w292) -> ()
            }
          }
        }
        "Array of VISA refnum" <- w248
        "Serial" <- w247
        "Array of Baud Rates" <- w246
        n226 = local read "term"() -> (w258:string)
        n227 = Concatenate Strings(w258, "Test des ports séries utilisés :\n" ("string")) -> (w259:string)
        n228 = local write "term"(w259) -> ()
        n229 = call <vilib>:"Close Config Data.vi"("error in (no error)"=w252, "refnum"=w254) -> ("error out"=→"config error out":errorcluster)  [unwired: 8 in, 1 out]
      }
      frame #10 {
        w410 = "communications" ("section")
        n230 = local read "Array of Files"() -> (w420:path[])
        n231 = Index Array(array=w420, index=0) -> (element=w419:path)
        n232 = call <vilib>:"Open Config Data.vi"("configuration file path"=w419) -> ("error out"=w411:errorcluster, "refnum"=w412:T3)  [unwired: 8 in, 1 out]
        n233 = call-poly <vilib>:"Read Key.vi"("section"=w410, "error in (no error)"=w411, "key"="TCS-IP", "refnum"=w412) -> ("error out"=w413:errorcluster, "value"=w407:string, "refnum out"=w414:T3)  [unwired: 4 in, 1 out]
        n234 = call-poly <vilib>:"Read Key.vi"("section"=w410, "error in (no error)"=w413, "key"="TCS-PN", "refnum"=w414) -> ("error out"=w398:errorcluster, "value"=w406:u32, "refnum out"=w399:T3)  [unwired: 4 in, 1 out]
        n235 = To Unsigned Word Integer(number=w406) -> (unsigned 16bit integer=w405:u16)
        n236 = call <vilib>:"Close Config Data.vi"("error in (no error)"=w398, "refnum"=w399) -> ()  [unwired: 8 in, 2 out]
        n237 = local read "term"() -> (w416:string)
        n238 = Concatenate Strings(w416, "Vérification du lien TCP/IP avec TCS ... " ("string")) -> (w417:string)
        n239 = TCP Open Connection(address=w407, remote port or service name=w405, timeout ms (60000)=3000) -> (connection ID=w404:refnum<k5>, error out=w394:errorcluster)  [unwired: 2 in]
        n240 = local write "term"(w417) -> ()
        n241 = Unbundle By Name(w394) -> ("status"=w401:bool)
        n242 = Type Cast(type="", x=w404) -> (*(type *) &x=w402:string)
        n243 = Not(x=w401) -> (.not. x?=w396:bool)
        "TCS" <- w396
        n244 = Type Cast(type=refnum<visa-resource-name> "-1" ("Table VRN"), x=w402) -> (*(type *) &x=w395:refnum<visa-resource-name>)
        n245 = case shown="Faux" w396 {
          selector: w396 -> [w421 _]
          frame False {
            n246 = local write "Go on ?"(w421) -> ()
          }
          frame True {
          }
        }
        n247 = call-poly "PolyCommError.vi"("VISA IN"=w395, "error IN"=w394) -> ("VISA OUT"=w393:refnum<visa-resource-name>, "error OUT"=w390:errorcluster)  [unwired: 11 in, 1 out]
        "TCS-CommVRN" <- w393
        n248 = local read "Array of VISA refnum"() -> (w392:refnum<visa-resource-name>[])
        n249 = Build Array (concatenate)(w392, w393) -> (w391:refnum<visa-resource-name>[])
        n250 = local write "Array of VISA refnum"(w391) -> ()
        n251 = local write "TCP Error"(w390) -> ()
      }
      frame #11 {
        n252 = local read "TCS"() -> (w422:bool)
        n253 = Select(t="OK!\n" ("string"), s=w422, f="Erreur!\n" ("string")) -> (s? t:f=w425:string)
        n254 = local read "term"() -> (w426:string)
        n255 = Concatenate Strings(w426, w425) -> (w427:string)
        n256 = local write "term"(w427) -> ()
      }
      frame #12 {
        w455 = "communications" ("section")
        n257 = local read "Array of Files"() -> (w462:path[])
        n258 = Index Array(array=w462, index=0) -> (element=w461:path)
        n259 = call <vilib>:"Open Config Data.vi"("configuration file path"=w461) -> ("error out"=w456:errorcluster, "refnum"=w457:T3)  [unwired: 8 in, 1 out]
        n260 = call-poly <vilib>:"Read Key.vi"("section"=w455, "error in (no error)"=w456, "key"="PRAMMS-IP", "refnum"=w457) -> ("error out"=w458:errorcluster, "value"=w446:string, "refnum out"=w459:T3)  [unwired: 4 in, 1 out]
        n261 = local read "Array of Folders"() -> (w432:path[])
        n262 = call-poly <vilib>:"Read Key.vi"("section"=w455, "error in (no error)"=w458, "key"="PRAMMS-PN", "refnum"=w459) -> ("error out"=w448:errorcluster, "value"=w452:u32, "refnum out"=w449:T3)  [unwired: 4 in, 1 out]
        n263 = Index Array(array=w432, index=0) -> (element=w430:path)
        n264 = call <vilib>:"Close Config Data.vi"("error in (no error)"=w448, "refnum"=w449) -> ()  [unwired: 8 in, 2 out]
        n265 = To Unsigned Word Integer(number=w452) -> (unsigned 16bit integer=w445:u16)
        n266 = Build Path(base path=w430, name or relative path="command.ini") -> (appended path=w428:path)
        n267 = call "SAOMM-connect.vi"("IP"=w446, "Port"=w445, "Signature"=u32 1886544237, "Command.ini"=w428) -> ("connection ID"=w444:refnum<k5>, "Connexion"=w443:bool, "Lecture"=w442:bool, "Écriture"=w441:bool, "Error OUT"=w438:errorcluster)  [unwired: 7 in]
        n268 = local read "term"() -> (w464:string)
        n269 = Concatenate Strings(w464, "Vérification du lien avec PRAMMS ... " ("string")) -> (w465:string)
        n270 = local write "term"(w465) -> ()
        n271 = Type Cast(type="", x=w444) -> (*(type *) &x=w450:string)
        n272 = Compound Arithmetic op=AND(w443, w442, w441) -> (w440:bool)
        "PRAMMS" <- w440
        n273 = Type Cast(type=refnum<visa-resource-name> "-1" ("Table VRN"), x=w450) -> (*(type *) &x=w437:refnum<visa-resource-name>)
        n274 = call-poly "PolyCommError.vi"("VISA IN"=w437, "error IN"=w438) -> ("VISA OUT"=w433:refnum<visa-resource-name>, "error OUT"=w436:errorcluster)  [unwired: 11 in, 1 out]
        "PRAMMS VRN" <- w433
        n275 = case shown="Faux" w440 {
          selector: w440 -> [w466 _]
          frame False {
            n276 = local write "Go on ?"(w466) -> ()
          }
          frame True {
          }
        }
        n277 = local read "Array of VISA refnum"() -> (w435:refnum<visa-resource-name>[])
        n278 = Build Array (concatenate)(w435, w433) -> (w434:refnum<visa-resource-name>[])
        n279 = local write "Array of VISA refnum"(w434) -> ()
      }
      frame #13 {
        n280 = local read "PRAMMS"() -> (w467:bool)
        n281 = Select(t="OK!\n" ("string"), s=w467, f="Erreur!\n" ("string")) -> (s? t:f=w470:string)
        n282 = local read "term"() -> (w471:string)
        n283 = Concatenate Strings(w471, w470) -> (w472:string)
        n284 = local write "term"(w472) -> ()
      }
      frame #14 {
        w499 = "communications" ("section")
        n285 = local read "Array of Files"() -> (w506:path[])
        n286 = Index Array(array=w506, index=0) -> (element=w505:path)
        n287 = call <vilib>:"Open Config Data.vi"("configuration file path"=w505) -> ("error out"=w500:errorcluster, "refnum"=w501:T3)  [unwired: 8 in, 1 out]
        n288 = call-poly <vilib>:"Read Key.vi"("section"=w499, "error in (no error)"=w500, "key"="PRAMMS-IP", "refnum"=w501) -> ("error out"=w502:errorcluster, "value"=w490:string, "refnum out"=w503:T3)  [unwired: 4 in, 1 out]
        n289 = local read "Array of Folders"() -> (w477:path[])
        n290 = call-poly <vilib>:"Read Key.vi"("section"=w499, "error in (no error)"=w502, "key"="PRAMMS-PN", "refnum"=w503) -> ("error out"=w492:errorcluster, "value"=w496:u32, "refnum out"=w493:T3)  [unwired: 4 in, 1 out]
        n291 = Index Array(array=w477, index=0) -> (element=w475:path)
        n292 = To Unsigned Word Integer(number=w496) -> (unsigned 16bit integer=w489:u16)
        n293 = Build Path(base path=w475, name or relative path="command.ini") -> (appended path=w473:path)
        n294 = call <vilib>:"Close Config Data.vi"("error in (no error)"=w492, "refnum"=w493) -> ()  [unwired: 8 in, 2 out]
        n295 = local read "term"() -> (w508:string)
        n296 = Concatenate Strings(w508, "Vérification du lien avec l'Hexapode ... " ("string")) -> (w509:string)
        n297 = local write "term"(w509) -> ()
        n298 = call "Hexapod-connect.vi"("IP"=w490, "Port"=w489, "Signature"=u32 1886544237, "path_config"=w473) -> ("connection ID"=w488:refnum<k5>, "Connexion"=w487:bool, "Lecture"=w486:bool, "Écriture"=w485:bool, "Error OUT"=w483:errorcluster)  [unwired: 7 in]
        n299 = Type Cast(type="", x=w488) -> (*(type *) &x=w494:string)
        n300 = Compound Arithmetic op=AND(w487, w486, w485) -> (w481:bool)
        "Hexapode" <- w481
        n301 = Type Cast(type=refnum<visa-resource-name> "-1" ("Table VRN"), x=w494) -> (*(type *) &x=w482:refnum<visa-resource-name>)
        n302 = call-poly "PolyCommError.vi"("VISA IN"=w482, "error IN"=w483) -> ("VISA OUT"=w478:refnum<visa-resource-name>, "error OUT"=w510:errorcluster)  [unwired: 11 in, 1 out]
        "Hexapod VRN" <- w478
        n303 = local read "Array of VISA refnum"() -> (w480:refnum<visa-resource-name>[])
        n304 = case shown="Faux" w481 {
          selector: w481 -> [w511 _]
          frame False {
            n305 = local write "Go on ?"(w511) -> ()
          }
          frame True {
          }
        }
        n306 = Build Array (concatenate)(w480, w478) -> (w479:refnum<visa-resource-name>[])
        n307 = local write "Array of VISA refnum"(w479) -> ()
      }
      frame #15 {
        n308 = local read "Hexapode"() -> (w512:bool)
        n309 = Select(t="OK!\n" ("string"), s=w512, f="Erreur!\n" ("string")) -> (s? t:f=w515:string)
        n310 = local read "term"() -> (w516:string)
        n311 = Concatenate Strings(w516, w515) -> (w517:string)
        n312 = local write "term"(w517) -> ()
      }
      frame #16 {
        n313 = flat-sequence {
          tunnel: [w532] -> w526
          tunnel: [w530] -> w525
          tunnel: [w533] -> w523
          tunnel: [w532] -> w522
          tunnel: [w530] -> w519
          tunnel: w526 -> [w552]
          tunnel: w525 -> [w551]
          tunnel: [w550] -> w524
          tunnel: w523 -> [_]
          tunnel: w522 -> [w549]
          tunnel: [w549] -> w521
          tunnel: [w548] -> w520
          tunnel: w519 -> [w547]
          tunnel: [w547] -> w518
          tunnel: w524 -> [w558]
          tunnel: w521 -> [w559]
          tunnel: w520 -> [w555]
          tunnel: w518 -> [w557]
          frame #0 {
            w538 = "communications" ("section")
            n314 = local read "Array of Files"() -> (w529:path[])
            n315 = Index Array(array=w529, index=0) -> (element=w527:path)
            n316 = call <vilib>:"Open Config Data.vi"("configuration file path"=w527) -> ("error out"=w539:errorcluster, "refnum"=w540:T3)  [unwired: 8 in, 1 out]
            n317 = call-poly <vilib>:"Read Key.vi"("section"=w538, "error in (no error)"=w539, "key"="cRIO-PN" ("section"), "refnum"=w540) -> ("error out"=w541:errorcluster, "value"=w531:u32, "refnum out"=w542:T3)  [unwired: 4 in, 1 out]
            n318 = To Unsigned Word Integer(number=w531) -> (unsigned 16bit integer=w530:u16)
            n319 = local read "term"() -> (w544:string)
            n320 = call-poly <vilib>:"Read Key.vi"("section"=w538, "error in (no error)"=w541, "key"="cRIO-IP" ("section"), "refnum"=w542) -> ("error out"=w534:errorcluster, "value"=w532:string, "refnum out"=w535:T3)  [unwired: 4 in, 1 out]
            n321 = Concatenate Strings(w544, "Connexion à la station météo ... " ("string")) -> (w545:string)
            n322 = local write "term"(w545) -> ()
            n323 = call <vilib>:"Close Config Data.vi"("error in (no error)"=w534, "refnum"=w535) -> ("error out"=w533:errorcluster)  [unwired: 8 in, 1 out]
          }
          frame #1 {
            n324 = TCP Open Connection(address=w552, remote port or service name=w551, timeout ms (60000)=3000) -> (connection ID=w548:refnum<k5>, error out=w554:errorcluster)  [unwired: 2 in]
            n325 = Unbundle By Name(w554) -> ("status"=w553:bool)
            n326 = Not(x=w553) -> (.not. x?=w550:bool)
          }
          frame #2 {
            n327 = case shown="Faux" w558 {
              tunnel: w555 -> [_ _]
              frame False {
                n328 = local read "term"() -> (w564:string)
                n329 = Concatenate Strings(w564, "Erreur!\n" ("string")) -> (w563:string)
                n330 = local write "Go on ?"(FALSE) -> ()
                n331 = local write "term"(w563) -> ()
              }
              frame True {
                n332 = local read "term"() -> (w567:string)
                n333 = Concatenate Strings(w567, "OK!\n" ("string")) -> (w566:string)
                n334 = local write "term"(w566) -> ()
              }
            }
            n335 = disable-structure shown="Disabled" {
              disable-tunnel: w555 -> [w561 _]
              frame Disabled {
                n336 = TCP Close Connection(connection ID=w561) -> (error out=→"TCP Error":errorcluster)  [unwired: 2 in, 1 out]
              }
              frame Enabled {
              }
            }
            n337 = Bundle("value"=w559, w557, "connection ID"=w555, w558) -> (w556:T4)  [unwired: 1 in]
            n338 = local write "Bundle-Meteo"(w556) -> ()
          }
        }
      }
      frame #17 {
        w592 = "chemins"
        n339 = local read "Array of Files"() -> (w577:path[])
        n340 = Index Array(array=w577, index=0) -> (element=w578:path)
        n341 = call <vilib>:"Open Config Data.vi"("configuration file path"=w578) -> ("error out"=w595:errorcluster, "refnum"=w596:T3)  [unwired: 8 in, 1 out]
        n342 = call-poly <vilib>:"Read Key.vi"("section"=w592, "error in (no error)"=w595, "key"="wgetexec", "refnum"=w596) -> ("error out"=w597:errorcluster, "value"=w574:path, "refnum out"=w598:T3)  [unwired: 4 in, 1 out]
        n343 = flat-sequence {
          tunnel: w574 -> [w624]
          tunnel: [w623] -> w587
          tunnel: [w622] -> w569
          tunnel: w589 -> [w627]
          tunnel: [w626] -> w588
          tunnel: [w625] -> w570
          frame #0 {
            n344 = File/Directory Info(path=w624) -> (error out=w623:errorcluster, resolved path=w622:path)  [unwired: 1 in, 5 out]
          }
          frame #1 {
            n345 = File/Directory Info(path=w627) -> (error out=w626:errorcluster, resolved path=w625:path)  [unwired: 1 in, 5 out]
          }
        }
        n346 = call-poly <vilib>:"Read Key.vi"("section"=w592, "error in (no error)"=w597, "key"="idlexec", "refnum"=w598) -> ("error out"=w593:errorcluster, "value"=w589:path, "refnum out"=w594:T3)  [unwired: 4 in, 1 out]
        n347 = local read "term"() -> (w582:string)
        n348 = Concatenate Strings(w582, "Vérification de l'existence des applications externes ... " ("string")) -> (w583:string)
        n349 = call <vilib>:"Close Config Data.vi"("error in (no error)"=w593, "refnum"=w594) -> ("error out"=→"error out":errorcluster, "file path"=w575:path)  [unwired: 8 in]
        n350 = local write "term"(w583) -> ()
        n351 = Unbundle By Name(w587) -> ("status"=w585:bool)
        n352 = Unbundle By Name(w588) -> ("status"=w586:bool)
        n353 = Not(x=w586) -> (.not. x?=w584:bool)
        n354 = Not(x=w585) -> (.not. x?=w576:bool)
        n355 = local write "wget"(w576) -> ()
        n356 = local write "IDL"(w584) -> ()
        n357 = case shown="Vrai" w576 {
          tunnel: w575 -> [_ w608]
          tunnel: w574 -> [_ w610]
          tunnel: [path "" w607] -> w571
          frame False {
          }
          frame True {
            n358 = local read "Array of Folders"() -> (w605:path[])
            n359 = call "Get_properties.vi"("Keyword"="queuelib" ("Section"), "Section"="chemins", "properties.ini"=w608) -> ("string"=w611:string)  [unwired: 6 in, 2 out]
            n360 = Index Array(array=w605, index=2) -> (element=w604:path)
            n361 = Path To String(path=w610) -> (string=w601:string)
            n362 = Concatenate Strings(w601, " --timeout=5 --tries=1" ("string"), " --http-user=carpe", " --http-password=noctem ", w611) -> (w612:string)
            "concatenated string" <- w612
            n363 = call <vilib>:"System Exec.vi"("run minimized? (F)"=TRUE, "working directory"=w604, "command line"=w612) -> ("error out"=w609:errorcluster, "standard error"=→"standard error":string, "standard output"=→"standard output":string)  [unwired: 5 in, 1 out]
            n364 = case shown="Erreur" w609 {
              tunnel: w604 -> [w620 _]
              tunnel: [w618 path ""] -> w607
              frame No Error {
                n365 = Build Path(base path=w620, name or relative path="table_technicien.dat") -> (appended path=w618:path)
              }
              frame Error {
              }
            }
          }
        }
        n366 = local read "Array of Files"() -> (w572:path[])
        n367 = Build Array (concatenate)(w572, w571, w570, w569) -> (w573:path[])
        n368 = local write "Array of Files"(w573) -> ()
      }
      frame #18 {
        n369 = local read "wget"() -> (w634:bool)
        n370 = local read "IDL"() -> (w635:bool)
        n371 = And(x=w635, y=w634) -> (x .and. y?=w628:bool)
        n372 = Select(t="OK!\n" ("string"), s=w628, f="Erreur!\n" ("string")) -> (s? t:f=w629:string)
        n373 = case shown="Faux" w628 {
          selector: w628 -> [w636 _]
          frame False {
            n374 = local write "Go on ?"(w636) -> ()
          }
          frame True {
          }
        }
        n375 = local read "term"() -> (w633:string)
        n376 = Concatenate Strings(w633, w629) -> (w632:string)
        n377 = local write "term"(w632) -> ()
      }
      frame #19 {
        # "VIs requierant une référence ou dont la face avant doit être caché"
        n378 = for {
          tunnel: string[] ["GUI\\CameraTuning.vi", "GUI\\Mode sync(pop-up).vi", "GUI\\InstrChoice.vi"] -> [w663] mode=indexing
          tunnel: [w658] -> w638 mode=indexing
          tunnel: [w657] -> w637 mode=indexing
          i -> [w652]
          n379 = local read "Array of Folders"() -> (w656:path[])
          n380 = Index Array(array=w656, index=4) -> (element=w655:path)
          n381 = Build Path(base path=w655, name or relative path=w663) -> (appended path=w662:path)
          n382 = Open VI Reference(vi path=w662) -> (vi reference=w653:refnum<vi>, error out=w651:errorcluster)  [unwired: 5 in]
          n383 = case shown="0" w652 {
            tunnel: w653 -> [_ w665 _ _]
            tunnel: w651 -> [_ w664 _ _]
            frame -1, Default {
            }
            frame 0 {
              n384 = case shown="Pas d'erreur" w664 {
                tunnel: w665 -> [w666 _]
                frame No Error {
                  n385 = global write "Globals.vi" "CameraTuning VI Refnum"(w666) -> ()
                }
                frame Error {
                }
              }
            }
            frame 1 {
            }
            frame 2 {
            }
          }
          n386 = property class="VI"(reference=w653, error in=w651) -> (reference out=w660:refnum<vi>, error out=w659:errorcluster, "Front Panel.Open"=w661:bool)
          n387 = case shown="Vrai" w661 {
            tunnel: w660 -> [w668 w673]
            tunnel: [w668 w672] -> w658
            tunnel: w659 -> [w667 w670]
            tunnel: [w667 w669] -> w657
            frame False {
            }
            frame True {
              n388 = property class="VI"(reference=w673, error in=w670, "Front Panel.Open"=FALSE) -> (reference out=w672:refnum<vi>, error out=w669:errorcluster)
            }
          }
        }
        n389 = local read "term"() -> (w640:string)
        n390 = Concatenate Strings(w640, "Vérification de l'état des sous-vis ... " ("string")) -> (w641:string)
        n391 = local write "term"(w641) -> ()
        n392 = flat-sequence {
          tunnel: w638 -> [_]
          tunnel: w637 -> [w646]
          frame #0 {
            n393 = for {
              tunnel: w646 -> [w650] mode=indexing
              tunnel: [w649] -> w645 mode=indexing
              n394 = Unbundle By Name(w650) -> ("status"=w649:bool)
            }
            n395 = disable-structure shown="Disabled" {
              frame Disabled {
                n396 = Wait (ms)(milliseconds to wait=u32 500) -> ()  [unwired: 1 out]
              }
              frame Enabled {
              }
            }
            n397 = Boolean Array To Number(Boolean array=w645) -> (number=w644:u32)
            n398 = Greater Than 0?(x=w644) -> (x > 0?=w643:bool)
            n399 = case shown="Vrai" w643 {
              frame False {
              }
              frame True {
                w648 = FALSE
                n400 = local write "Go on ?"(w648) -> ()
                n401 = local write "SubVIs"(w648) -> ()
              }
            }
          }
        }
      }
      frame #20 {
        n402 = local read "SubVIs"() -> (w674:bool)
        n403 = Select(t="OK!\n" ("string"), s=w674, f="Erreur!\n" ("string")) -> (s? t:f=w677:string)
        n404 = local read "term"() -> (w678:string)
        n405 = Concatenate Strings(w678, w677) -> (w679:string)
        n406 = local write "term"(w679) -> ()
      }
      frame #21 {
        # "Mettre à la fin pour recommencer tout ..."
        n407 = local read "Go on ?"() -> (w683:bool)
        n408 = case shown="Faux" w683 {
          tunnel: [w713 FALSE ("true")] -> w684
          frame False {
            w712 = T2."Enabled" ("Disabled")
            n409 = disable-structure shown="Disabled" {
              disable-tunnel: [w714 TRUE ("true")] -> w713
              frame Disabled {
                n410 = One Button Dialog(message="Une ou plusieurs erreurs se sont produites lors de l'initialisation.\nVous pouvez annuler l'ouverture du programme, recommencez l'initialisation ou ignorer les erreurs.\n\nCependant, si vous ignorez les erreurs, il se peut que \ncertaines fonctionnalités ne soient pas disponibles") -> (true=w714:bool)  [unwired: 1 in]
              }
              frame Enabled {
              }
            }
            n411 = property on="cancel" class="Bool"("DisabledEnum"=w712) -> ()  [unwired: 2 in, 2 out]
            n412 = property on="ignore" class="Bool"("DisabledEnum"=w712) -> ()  [unwired: 2 in, 2 out]
            n413 = property on="restart" class="Bool"("DisabledEnum"=w712) -> ()  [unwired: 2 in, 2 out]
          }
          frame True {
          }
        }
        n414 = local read "term"() -> (w680:string)
        n415 = case shown="Vrai" w684 {
          tunnel: [u32 0 w694] -> w682
          tunnel: w680 -> [_ w693]
          frame False {
            (unwired) TRUE
          }
          frame True {
            n416 = while {
              tunnel: [w705] -> w694
              tunnel: w693 -> [w701]
              i -> [w704]
              stop <- w707 stop-if-true
              n417 = Build Array("cancel", "restart", "ignore") -> (w706:bool[])
              n418 = Quotient & Remainder(x=w704, y=10) -> (x-y*floor(x/y)=w697:i32)  [unwired: 1 out]
              n419 = Boolean Array To Number(Boolean array=w706) -> (number=w705:u32)
              n420 = Less?(x=w697, y=6) -> (x < y?=w696:bool)
              n421 = Wait (ms)(milliseconds to wait=u32 100) -> ()  [unwired: 1 out]
              n422 = Greater Than 0?(x=w705) -> (x > 0?=w707:bool)
              n423 = Select(t="\nEn attente de la réponse de l'usagé ..." ("string"), s=w696, f="") -> (s? t:f=w699:string)
              n424 = Concatenate Strings(w701, w699) -> (w700:string)
              n425 = local write "term"(w700) -> ()
            }
          }
        }
        n426 = case shown="2" w682 {
          tunnel: [TRUE TRUE FALSE TRUE] -> w681
          frame 0, Default {
          }
          frame 1 {
            n427 = local write "Go on ?"(FALSE ("Go on ?")) -> ()
          }
          frame 2 {
            n428 = local write "Go on ?"(FALSE ("Go on ?")) -> ()
          }
          frame 4 {
            n429 = local write "Go on ?"(TRUE ("Go on ?")) -> ()
          }
        }
      }
      frame #22 {
        n430 = local read "Go on ?"() -> (w719:bool)
        n431 = case shown="Vrai" w719 {
          tunnel: w718 -> [_ w723]
          frame False {
          }
          frame True {
            n432 = Concatenate Strings(w723, "\nVérifications complétées\nBonne Nuit !!!" ("string")) -> (w722:string)
            n433 = local write "term"(w722) -> ()
            n434 = disable-structure shown="Enabled" {
              frame Disabled {
                n435 = Wait (ms)(milliseconds to wait=u32 666) -> ()  [unwired: 1 out]
              }
              frame Enabled {
                n436 = Wait (ms)(milliseconds to wait=u32 200) -> ()  [unwired: 1 out]
              }
              frame Disabled {
              }
            }
            "SkipInstr" <- "SkipInstr"
          }
        }
      }
    }
  }
  n437 = disable-structure shown="Disabled" {
    frame Disabled {
      n438 = flat-sequence {
        tunnel: w743 -> [w746]
        tunnel: [w746] -> w726
        frame #0 {
          n439 = Wait (ms)(milliseconds to wait=u32 500) -> ()  [unwired: 1 out]
        }
      }
      n440 = call "MC-BonOMM_talker.vi"("MC-BonOMM VRN"=w726, "Commande"="m", "byte count"=u32 1, "Timeout (ms)"=3000, "answer=command?"=FALSE) -> ("Answer"=w728:string, "ok ?"=w729:bool)
      n441 = VISA Write(write buffer="r" ("Commande")) -> (VISA resource name out=w741:refnum<visa-resource-name>)  [unwired: 2 in, 2 out]
      n442 = property class="Instr"(reference=w741) -> (reference out=w740:refnum<visa-resource-name>, "Serial Settings:Number of Bytes at Serial Port"=w739:u32)  [unwired: 1 in, 1 out]
      n443 = Equal?(x="f", y=w728) -> (x = y?=w733:bool)
      n444 = Equal?(x=w728, y="x") -> (x = y?=w734:bool)
      n445 = Or(x=w733, y=w734) -> (x .or. y?=w730:bool)
      n446 = And(x=w730, y=w729) -> (x .and. y?=w727:bool)
      n447 = VISA Read(VISA resource name=w740, byte count=w739) -> (VISA resource name out=w743:refnum<visa-resource-name>)  [unwired: 1 in, 3 out]
      n448 = case shown="Vrai" w727 {
        tunnel: [w747 w761] -> w744
        tunnel: w743 -> [_ w752]
        frame False {
          n449 = Two Button Dialog(message="MC-BonOMM n'a pas été détecté !\nSouhaitez-vous recommencer l'initalisation ?", 1:"NON" ("F button name (\"Cancel\")"), 2:"OUI" ("T button name (\"OK\")")) -> (T button?=w748:bool)
          n450 = Not(x=w748) -> (.not. x?=w747:bool)
        }
        frame True {
          n451 = call <vilib>:"Three Button Dialog.vi"("Allow user to close window? (TRUE)"=FALSE, "Justify Message (Left)"=enum16{"Left", "Center", "Right"}."Center", "Right Button Text (\"Cancel\")"="Foyer ST-133" ("F button name (\"Cancel\")"), "Center Button Text (\"No\")"="RàF (PANO-II)" ("F button name (\"Cancel\")"), "Left Button Text (\"Yes\")"="RàF (BonOMM)" ("T button name (\"OK\")"), "message"="MC-BonOMM a été détecté !\nQuel mode souhaité vous utiliser ?") -> ("Which Button?"=w754:T5)  [unwired: 5 in]
          n452 = case shown="\"Left Button\", Par défaut" w754 {
            tunnel: ["o" "x" "f"] -> w753
            frame "Center Button" {
            }
            frame "Right Button" {
            }
            frame "Left Button", Default {
            }
          }
          n453 = call "MC-BonOMM_talker.vi"("MC-BonOMM VRN"=w752, "Commande"=w753, "Timeout (ms)"=1000, "answer=command?"=TRUE) -> ("ok ?"=w761:bool)  [unwired: 1 in, 1 out]
        }
      }
    }
    frame Enabled {
    }
  }
